vi "TranslatorBooster.vi"() -> ()   [LabVIEW 2014, in "Complex Numbers.lvlib"]
uses:
  <vilib>/Aledyne-TSXperts/Arduino Compatible Compiler for LabVIEW/addons/Complex Numbers/Complex Numbers.lvlib
  <vilib>/regexp/Match Regular Expression.xnode
panel:
  in  "Output dir":path=path "C:/Program Files/National Instruments/LabVIEW 2014/vi.lib/Aledyne-TSXperts/Arduino Compatible Compiler for LabVIEW/addons/Complex Numbers/generated VIs"
  out "Func. output type":string[](array[string])
  out "Params":string[][](array[string])
  out "Func. params":string[](array[string])
  out "Function actual token":string
  out "Readed functions":string[](array[string])
  out "Function Name":string
  out "Function name reading":bool
  out "Class name found.":bool
  out "Functions beginning found.":bool
  out "Input header file.":string[](array[string])
  out "Class name":string
  out "Error Out":errorcluster
  in  "Error In":errorcluster
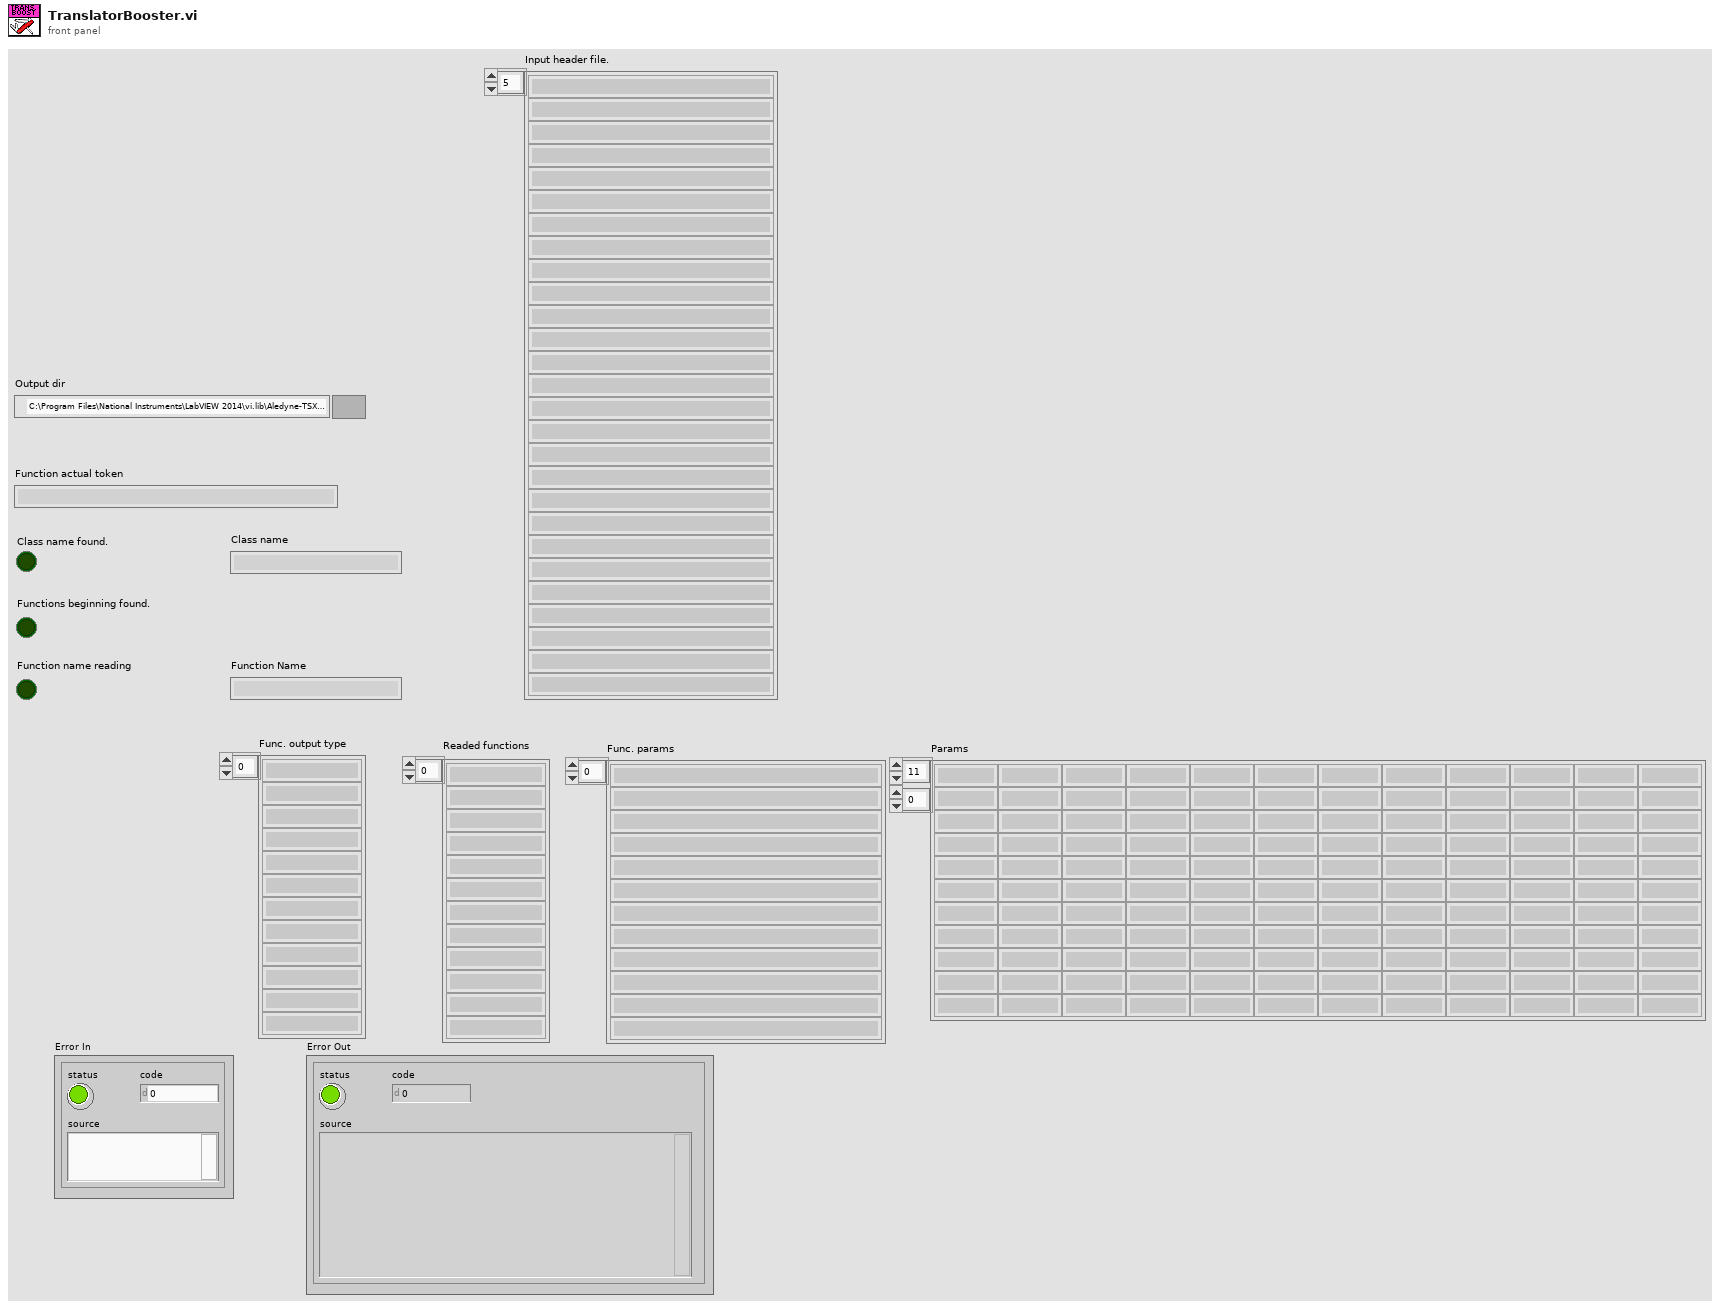
[diagram p1: front panel]
types:
  T1 = enum16{"open", "replace", "create", "open or create", "replace or create", "replace or create with confirmation"}
  T2 = cluster{"Function names":string[], "Function parameters":string[][], "Output types":string[]}
  T3 = enum32{"invalid lock state", "Not Locked", "Locked (No Password)", "Password-protected"}
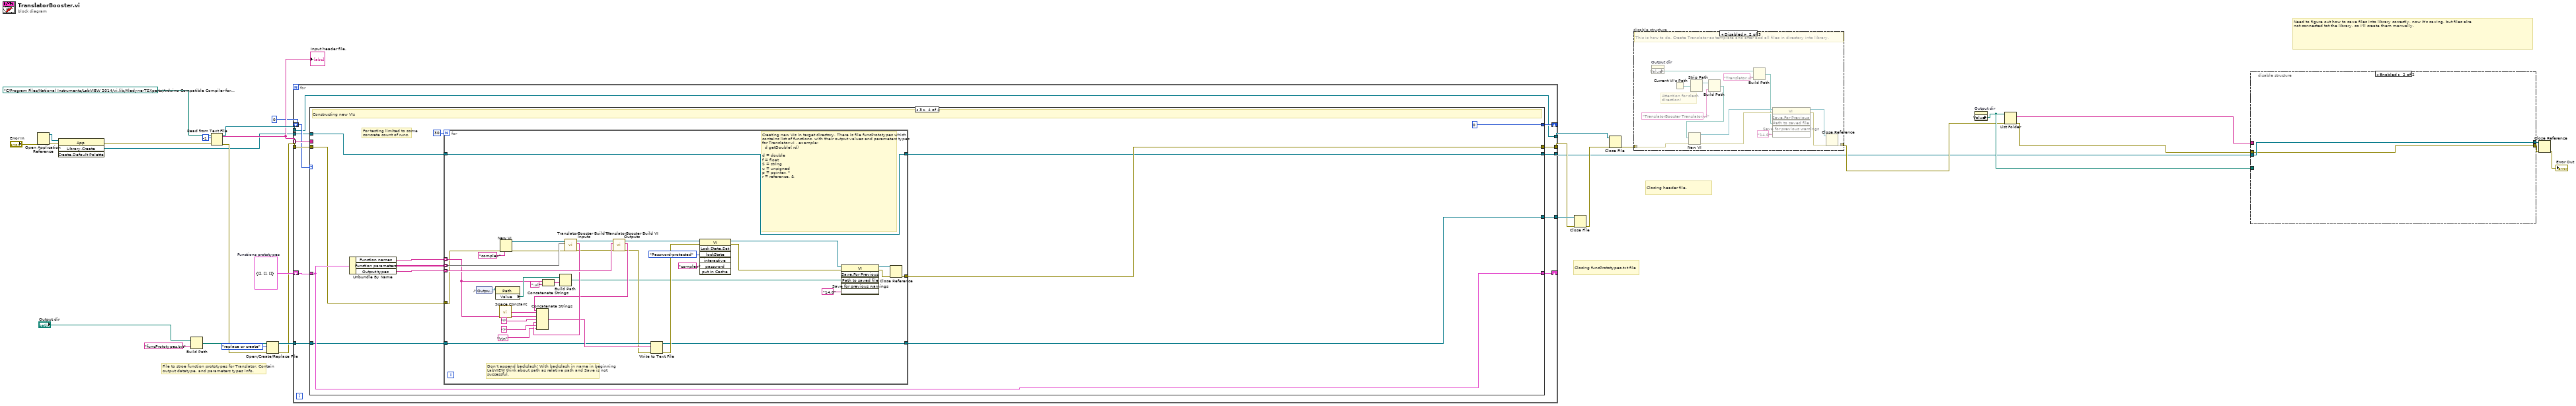
[diagram p0: block diagram]
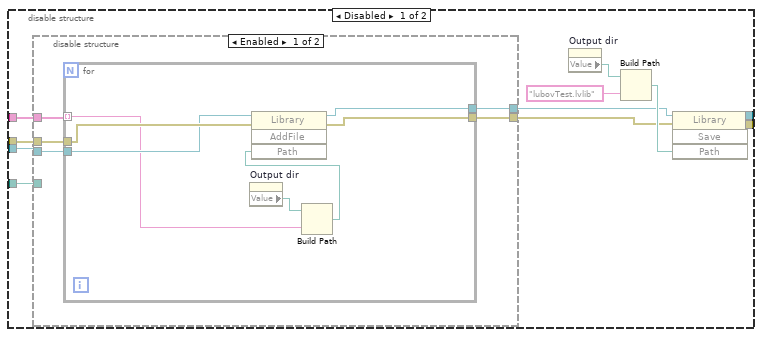
[diagram p2: hidden frame]
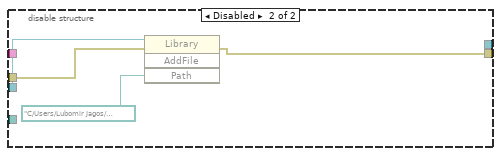
[diagram p3: hidden frame]
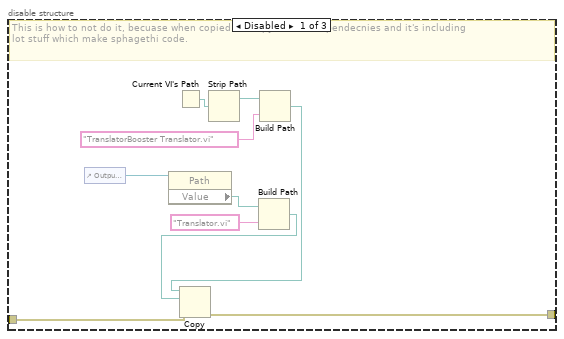
[diagram p4: hidden frame]
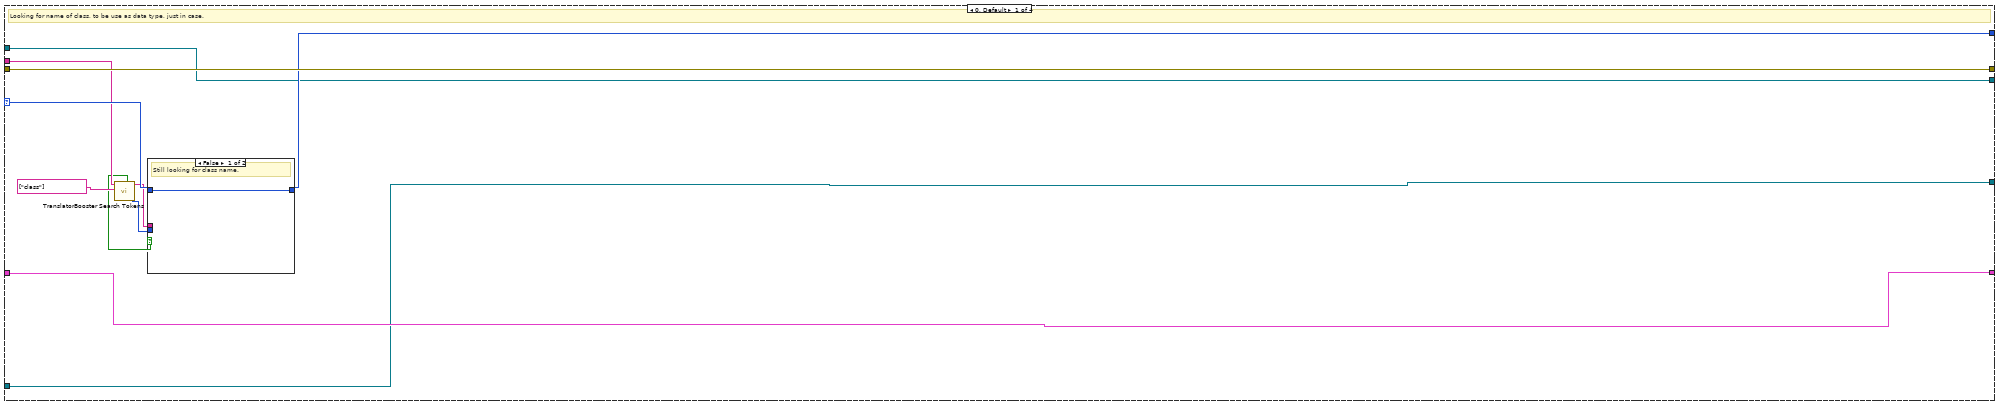
[diagram p6: hidden frame]
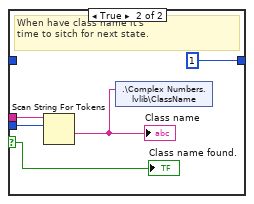
[diagram p7: hidden frame]
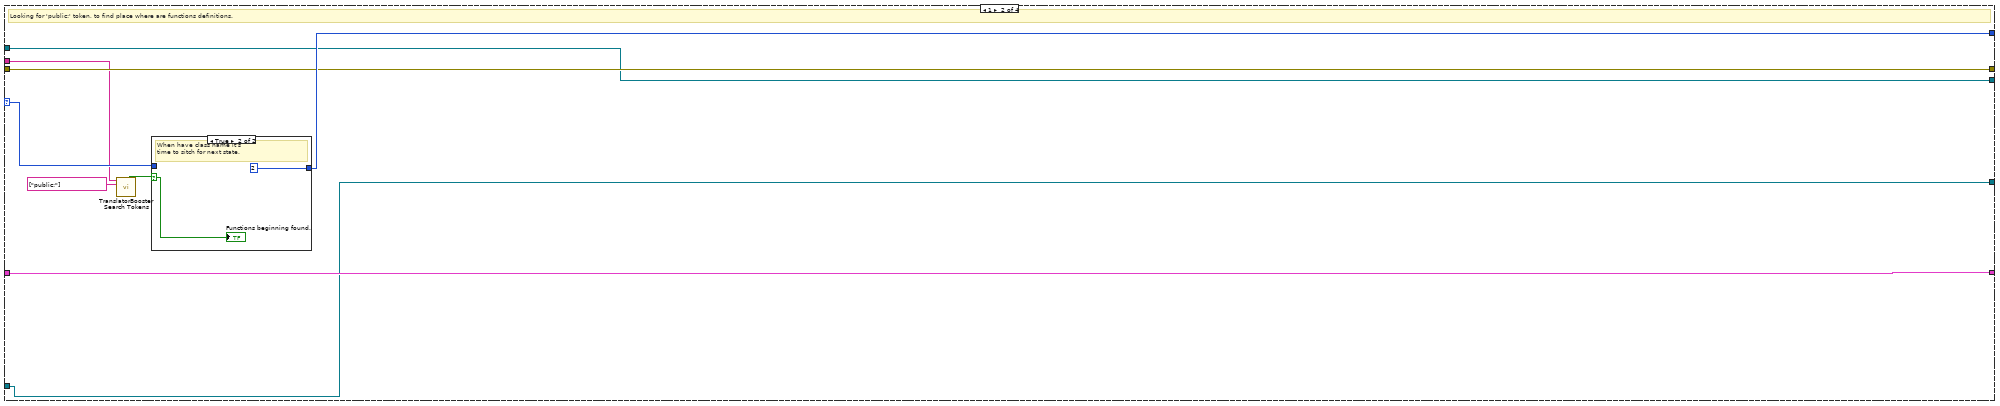
[diagram p8: hidden frame]
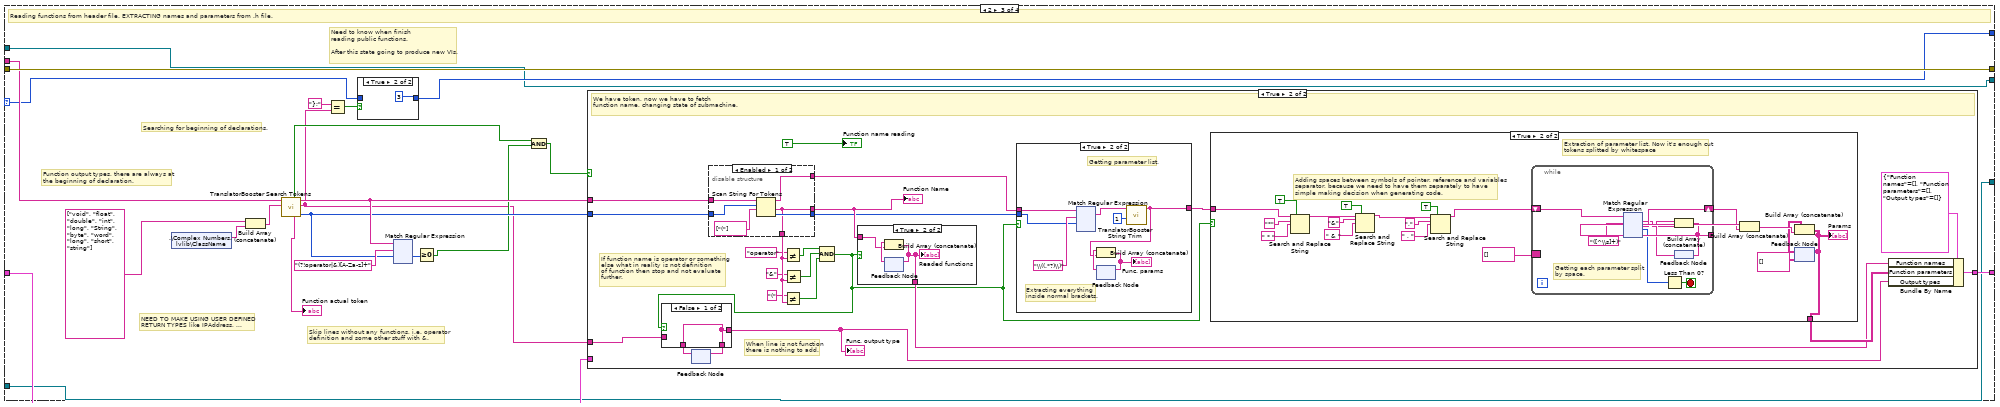
[diagram p10: hidden frame]
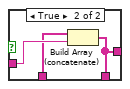
[diagram p13: hidden frame]
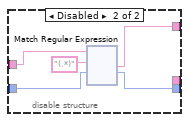
[diagram p16: hidden frame]
diagram:
  w25 = T2 {"Function names"=[], "Function parameters"=[], "Output types"=[]}  # Functions prototypes
  # "Need to figure out how to save files into library correctly, now it's saving, but files alre\nnot connected tot the library, so I'll create them manually."
  # "File to stroe function prototypes for Translator. Contain\noutput datatype, and parameters types info."
  # "Closing header file."
  # "Closing funcPrototypes.txt file"
  n1 = Open Application Reference(8:"Error In") -> (0:w12:errorcluster, 3:w11:refnum<vi>)  [unwired: 3 in]
  n2 = invoke class="App" method="Library.Create"(reference=w11, error in=w12) -> (error out=w9:errorcluster, "Create Library"=w10:refnum<vi>)  [unwired: 2 in, 2 out]
  n3 = Build Path(base path="Output dir", name or relative path="funcPrototypes.txt") -> (appended path=w18:path)
  n4 = Read from Text File(file (use dialog)=path "C:/Program Files/National Instruments/LabVIEW 2014/vi.lib/Aledyne-TSXperts/Arduino Compatible Compiler for LabVIEW/addons/Complex Numbers/libraries/____aux_complex.h", count=-1, error in=w9) -> (refnum out=w28:refnum<file>, text=w27:string[], error out=w17:errorcluster)  [unwired: 1 in, 1 out]
  "Input header file." <- w27
  n5 = Open/Create/Replace File(file path (use dialog)=w18, error in=w17, operation (0:open)=T1."replace or create") -> (refnum out=w23:refnum<file>, error out=w16:errorcluster)  [unwired: 3 in, 1 out]
  n6 = for {
    tunnel: [w38] -> w31
    tunnel: w16 -> [w42]
    tunnel: w28 -> [w38]
    tunnel: w27 -> [w43] mode=indexing
    tunnel: [w41] -> w21
    shift-right: [w40] -> _
    shift-left: 0 ("offset past token") -> [w39]
    shift-right: [w37] -> _
    shift-left: w25 -> [w36]
    tunnel: w23 -> [w35]
    tunnel: [w34] -> w22
    tunnel: w10 -> [w33]
    tunnel: [w32] -> w1
    n7 = case shown="3" w39 {
      selector: w39 -> [w53 w69 w79 _]
      tunnel: w43 -> [w50 w65 w93 _]
      tunnel: w42 -> [w54 w67 w94 w638]
      tunnel: [w54 w67 w94 w636] -> w41
      tunnel: [w52 w68 w78 0 ("offset past token")] -> w40
      tunnel: [w46 w63 w76 w641] -> w37
      tunnel: w36 -> [w46 w63 w75 w641]
      tunnel: w35 -> [w45 w62 w74 w635]
      tunnel: [w45 w62 w74 w634] -> w34
      tunnel: w33 -> [w44 w61 w73 w633]
      tunnel: [w44 w61 w73 w632] -> w32
      frame 0, Default {
        # "Looking for name of class, to be use as data type, just in case."
        n8 = call <vilib>:"TranslatorBooster Search Tokens.vi"("search tokens"=string[] ["class"] ("operators (none)"), "input string"=w50) -> ("offset past token"=w49:i32, "input string"=w47:string, "token found?"=w48:bool)  [unwired: 4 in, 3 out]
        n9 = case shown="False" w48 {
          selector: w48 -> [_ w57]
          tunnel: w49 -> [_ w60]
          tunnel: w47 -> [_ w59]
          tunnel: w53 -> [w55 _]
          tunnel: [w55 1 ("offset past token")] -> w52
          frame False {
            # "Still looking for class name."
          }
          frame True {
            # "When have class name it's\ntime to sitch for next state."
            n10 = Scan String For Tokens(8:w60, 9:w59) -> (1:w56:string)  [unwired: 4 in, 3 out]
            "Class name" <- w56
            n11 = shared-variable ".\\Complex Numbers.lvlib\\ClassName"(w56) -> ()  [unwired: 1 in, 1 out]
            "Class name found." <- w57
          }
        }
      }
      frame 1 {
        # "Looking for 'public:' token, to find place where are functions definitions."
        n12 = call <vilib>:"TranslatorBooster Search Tokens.vi"("search tokens"=string[] ["public:"] ("operators (none)"), "input string"=w65) -> ("token found?"=w64:bool)  [unwired: 4 in, 5 out]
        n13 = case shown="True" w64 {
          selector: w64 -> [_ w71]
          tunnel: [w70 2 ("offset past token")] -> w68
          tunnel: w69 -> [w70 _]
          frame False {
            # "Still looking for functions\nbeginning."
          }
          frame True {
            # "When have class name it's\ntime to sitch for next state."
            "Functions beginning found." <- w71
          }
        }
      }
      frame 2 {
        # "NEED TO MAKE USING USER DEFINED\nRETURN TYPES like IPAddress, ..."
        # "Function output types, there are always at\nthe beginning of declaration."
        # "Need to know when finish\nreading public functions.\n\nAfter this state going to produce new VIs."
        # "Searching for beginning of declarations."
        # "Skip lines without any functions, i.e. operator\ndefinition and some other stuff with &."
        # "Reading functions from header file. EXTRACTING names and parameters from .h file."
        n14 = shared-variable ".\\Complex Numbers.lvlib\\ClassName"() -> (w91:string)  [unwired: 1 in, 1 out]
        n15 = Build Array (concatenate)(string[] ["void", "float", "double", "int", "long", "String", "byte", "word", "long", "short", "string"] ("operators (none)"), w91) -> (w90:string[])
        n16 = call <vilib>:"TranslatorBooster Search Tokens.vi"("search tokens"=w90, "input string"=w93) -> ("offset past token"=w83:i32, "output token"=w77:string, "input string"=w86:string, "actual token"=→"Function actual token":string, "token found?"=w85:bool)  [unwired: 4 in, 1 out]
        n17 = Equal?(x="};", y=w77) -> (x = y?=w80:bool)
        n18 = case shown="True" w80 {
          tunnel: w79 -> [w95 _]
          tunnel: [w95 3 ("offset past token")] -> w78
          frame False {
          }
          frame True {
          }
        }
        n19 = xnode "Match Regular Expression"("input string"=w86, "regular expression"="(?!operator|&)[A-Za-z]+", "offset (0)"=w83) -> ("offset past match"=w88:i32)  [unwired: 3 in, 4 out]
        n20 = Greater Or Equal To 0?(x=w88) -> (x >= 0?=w82:bool)
        n21 = Compound Arithmetic op=AND(w85, w82) -> (w84:bool)
        n22 = case shown="True" w84 {
          tunnel: w86 -> [_ w233]
          tunnel: w83 -> [_ w232]
          tunnel: w77 -> [_ w215]
          tunnel: [w211 w216] -> w76
          tunnel: w75 -> [w211 _]
          frame False {
            # "Still looking for functions\nbeginning."
          }
          frame True {
            # "When line is not function\nthere is nothing to add."
            # "If function name is operator or something\nelse what in reality is not definition\nof function then stop and not evaluate\nfurther."
            # "We have token, now we have to fetch\nfunction name, changing state of submachine."
            n23 = feedback #1() -> (w213:string[])  [unwired: 1 in]
            n24 = disable-structure shown="Enabled" {
              disable-tunnel: w233 -> [w509 w514]
              disable-tunnel: w232 -> [w508 w510]
              disable-tunnel: [w506 w512] -> w231
              disable-tunnel: [w505 w511] -> w228
              disable-tunnel: [w504 _] -> w229
              disable-tunnel: [w504 _] -> w227
              frame Enabled {
                n25 = Scan String For Tokens(7:string[] ["("] ("operators (none)"), 8:w508, 9:w509) -> (0:w505:i32, 1:w504:string, 3:w506:string)  [unwired: 3 in, 1 out]
              }
              frame Disabled {
                n26 = xnode "Match Regular Expression"("input string"=w514, "regular expression"="(.*)", "offset (0)"=w510) -> ("after match"=w512:string, "offset past match"=w511:i32)  [unwired: 3 in, 3 out]
              }
            }
            "Function Name" <- w229
            n27 = Not Equal?(x="operator", y=w227) -> (x != y?=w223:bool)
            n28 = Not Equal?(x="(", y=w227) -> (x != y?=w221:bool)
            n29 = Not Equal?(x="&", y=w227) -> (x != y?=w222:bool)
            n30 = Compound Arithmetic op=AND(w223, w222, w221) -> (w212:bool)
            n31 = case shown="False" w212 {
              tunnel: w215 -> [_ w237]
              tunnel: [w235 w238] -> w219
              tunnel: [w235 w238] -> w214
              tunnel: w213 -> [w235 w236]
              frame False {
              }
              frame True {
                n32 = Build Array (concatenate)(w236, w237) -> (w238:string[])
              }
            }
            "Func. output type" <- w219
            n33 = feedback-in #1(w214) -> ()
            n34 = case shown="True" w212 {
              tunnel: w229 -> [_ w630]
              tunnel: [_ w629] -> w217
              frame False {
              }
              frame True {
                n35 = feedback #2() -> (w631:string[])  [unwired: 1 in]
                n36 = Build Array (concatenate)(w631, w630) -> (w629:string[])
                "Readed functions" <- w629
                n37 = feedback-in #2(w629) -> ()
              }
            }
            n38 = case shown="True" w212 {
              tunnel: w231 -> [w381 w389]
              tunnel: [w381 w386] -> w230
              tunnel: w228 -> [_ w383]
              frame False {
              }
              frame True {
                # "Extracting everything\ninside normal brackets."
                # "Getting parameter list."
                n39 = xnode "Match Regular Expression"("input string"=w389, "regular expression"="\\((.*?)\\)", "offset (0)"=w383) -> ("whole match"=w385:string)  [unwired: 3 in, 4 out]
                n40 = feedback #3() -> (w387:string[])  [unwired: 1 in]
                n41 = call <vilib>:"TranslatorBooster String Trim.vi"("Count"=u8 1, "String In"=w385) -> ("Trimmed String"=w386:string)  [unwired: 9 in]
                n42 = Build Array (concatenate)(w387, w386) -> (w382:string[])
                "Func. params" <- w382
                n43 = feedback-in #3(w382) -> ()
              }
            }
            n44 = case shown="True" w212 {
              tunnel: w230 -> [_ w246]
              tunnel: [_ w252] -> w220
              frame False {
              }
              frame True {
                # "Adding spaces between symbols of pointer, reference and variables\nseparator, because we need to have them separately to have\nsimple making decision when generating code."
                # "Extraction of parameter list. Now it's enough cut\ntokens splitted by whitespace"
                n45 = Search and Replace String(replace all?=TRUE ("replace all? (F)"), input string=w246, search string="*", replace string=" * " ("search string")) -> (result string=w251:string)  [unwired: 4 in, 3 out]
                n46 = Search and Replace String(replace all?=TRUE ("replace all? (F)"), input string=w251, search string="&", replace string=" & " ("search string")) -> (result string=w243:string)  [unwired: 4 in, 3 out]
                n47 = Search and Replace String(replace all?=TRUE ("replace all? (F)"), input string=w243, search string=",", replace string=" , " ("search string")) -> (result string=w242:string)  [unwired: 4 in, 3 out]
                n48 = while {
                  tunnel: [w265] -> w257
                  border: string[] [] -> [_]
                  shift-right: [w263] -> w254
                  shift-left: w242 -> [w259]
                  stop <- w266 stop-if-true
                  # "Getting each parameter split\nby space."
                  n49 = xnode "Match Regular Expression"("input string"=w259, "regular expression"="([^\\s]+)") -> ("whole match"=w260:string, "after match"=w263:string, "offset past match"=w262:i32)  [unwired: 4 in, 2 out]
                  n50 = Less Than 0?(x=w262) -> (x < 0?=w266:bool)
                  n51 = feedback #4() -> (w261:string[])
                  n52 = Build Array (concatenate)(w261, w260) -> (w265:string[])
                  n53 = feedback-in #4(w265) -> ()
                }
                n54 = Build Array (concatenate)(w257, w254) -> (w256:string[])
                n55 = feedback #5(string[][] []) -> (w255:string[][])
                n56 = Build Array (concatenate)(w255, w256) -> (w252:string[][])
                "Params" <- w252
                n57 = feedback-in #5(w252) -> ()
              }
            }
            n58 = Bundle By Name(cluster=T2 {"Function names"=[], "Function parameters"=[], "Output types"=[]} ("input cluster"), "Function names"=w217, "Function parameters"=w220, "Output types"=w219) -> (w216:T2)
            "Function name reading" <- TRUE ("Function return type reading")
          }
        }
      }
      frame 3 {
        # "For testing limited to some\nconcrete count of runs."
        # "Constructing new VIs"
        n59 = Unbundle By Name(w641) -> ("Function names"=w643:string[], "Function parameters"=w640:string[][], "Output types"=w639:string[])
        n60 = for {
          N: 30 -> [_]
          tunnel: w643 -> [w658] mode=indexing
          tunnel: w640 -> [w677] mode=indexing
          tunnel: w639 -> [w676] mode=indexing
          tunnel: w638 -> [w653]
          tunnel: [w652] -> w636
          tunnel: w635 -> [w666]
          tunnel: [w662] -> w634
          tunnel: w633 -> [w644]
          tunnel: [w644] -> w632
          # "Don't append backslash! With backslash in name in beginning\nLabVIEW think about path as relative path and Save is not\nsuccessful."
          # "Creating new VIs in target directory. There is file funcPrototypes which contains list of functions, with their output values and parameters types for Translator.vi , example:\n  d getDouble( rd)\n\nd = double\nf = float\nS = string\nu = unsigned\np = pointer, *\nr = reference, &"
          n61 = control-ref of="Output dir"() -> (w661:refnum<vi>)
          n62 = property class="Path"(reference=w661) -> ("Value"=w660:path)  [unwired: 1 in, 2 out]
          n63 = call <vilib>:"Space Constant.vi"() -> ("String"=w669:string)
          n64 = New VI(6:"complex" ("password"), 8:w653) -> (0:w656:errorcluster, 3:w648:refnum<vi>)  [unwired: 5 in]
          n65 = Concatenate Strings(w658, ".vi" ("string")) -> (w659:string)
          n66 = Build Path(base path=w660, name or relative path=w659) -> (appended path=w651:path)
          n67 = call <vilib>:"TranslatorBooster Build VI Inputs.vi"("error in (no error)"=w656, "Function parameters"=w677, "VI in"=w648) -> ("error out"=w655:errorcluster, "ParamsType abbr."=w670:string, "VI out"=w654:refnum<vi>)  [unwired: 6 in]
          n68 = call <vilib>:"TranslatorBooster Build VI Outputs.vi"("error in (no error)"=w655, "Output type"=w676, "VI in"=w654) -> ("error out"=w665:errorcluster, "OutputType abbr."=w668:string, "VI out"=w675:refnum<vi>)  [unwired: 6 in]
          n69 = Concatenate Strings(w668, w669, w658, "(" ("string"), w670, ")" ("string"), "\r\n") -> (w667:string)
          n70 = Write to Text File(file (use dialog)=w666, text=w667, error in=w665) -> (refnum out=w662:refnum<file>, error out=w664:errorcluster)  [unwired: 1 in, 1 out]
          n71 = invoke class="VI" method="Lock State.Set"(reference=w675, error in=w664, "lockState"=T3."Password-protected" ("Lock State"), "password"="complex" ("Password")) -> (reference out=w645:refnum<vi>, error out=w646:errorcluster)  [unwired: 3 in, 5 out]
          n72 = invoke class="VI" method="Save.For Previous"(reference=w645, error in=w646, "Path to saved file"=w651, "Oldest compatible target version"="14.0" ("Target Version")) -> (reference out=w650:refnum<vi>, error out=w649:errorcluster)  [unwired: 2 in, 4 out]
          n73 = Close Reference(reference=w650, error in (no error)=w649) -> (error out=w652:errorcluster)
        }
      }
    }
  }
  n74 = Close File(refnum=w22, error in=w21) -> (error out=w20:errorcluster)  [unwired: 1 out]
  n75 = Close File(refnum=w31, error in=w20) -> (error out=w14:errorcluster)  [unwired: 1 out]
  n76 = disable-structure shown="Disabled" {
    disable-tunnel: w14 -> [w688 w702 w703]
    disable-tunnel: [w679 w695 w703] -> w6
    frame Disabled {
      # "This is how to not do it, becuase when copied it's copy with all dependecnies and it's including\nlot stuff which make sphagethi code."
      n77 = control-ref of="Output dir"() -> (w682:refnum<vi>)
      n78 = property class="Path"(reference=w682) -> ("Value"=w681:path)  [unwired: 1 in, 2 out]
      n79 = Current VI's Path() -> (path=w687:path)
      n80 = Strip Path(path=w687) -> (stripped path=w686:path)  [unwired: 1 out]
      n81 = Build Path(base path=w681, name or relative path="Translator.vi") -> (appended path=w680:path)
      n82 = Build Path(base path=w686, name or relative path="TranslatorBooster Translator.vi") -> (appended path=w684:path)
      n83 = Copy(8:w688, 10:w680, 11:w684) -> (0:w679:errorcluster)  [unwired: 2 in, 2 out]
    }
    frame Disabled {
      # "Attention for slash\ndirection!"
      # "This is how to do. Create Translator as template and after add all files in directory into library."
      n84 = property on="Output dir" class="Path"() -> ("Value"=w691:path)  [unwired: 2 in, 2 out]
      n85 = Current VI's Path() -> (path=w689:path)
      n86 = Strip Path(path=w689) -> (stripped path=w690:path)  [unwired: 1 out]
      n87 = Build Path(base path=w690, name or relative path="TranslatorBooster Translator.vi") -> (appended path=w698:path)
      n88 = New VI(8:w702, 10:w698) -> (0:w700:errorcluster, 3:w701:refnum<vi>)  [unwired: 5 in]
      n89 = Build Path(base path=w691, name or relative path="Translator.vi") -> (appended path=w696:path)
      n90 = invoke class="VI" method="Save.For Previous"(reference=w701, error in=w700, "Path to saved file"=w696, "Oldest compatible target version"="14.0" ("Target Version")) -> (reference out=w693:refnum<vi>, error out=w694:errorcluster)  [unwired: 2 in, 4 out]
      n91 = Close Reference(reference=w693, error in (no error)=w694) -> (error out=w695:errorcluster)
    }
    frame Enabled {
    }
  }
  n92 = property on="Output dir" class="Path"() -> ("Value"=w7:path)  [unwired: 2 in, 2 out]
  n93 = List Folder(path=w7, error in=w6) -> (filenames=w8:string[], error out=w2:errorcluster)  [unwired: 2 in, 2 out]
  n94 = disable-structure shown="Enabled" {
    disable-tunnel: w8 -> [w714 _]
    disable-tunnel: w7 -> [w713 _]
    disable-tunnel: [w712 w733] -> w4
    disable-tunnel: [w711 w732] -> w3
    disable-tunnel: w2 -> [w710 w732]
    disable-tunnel: w1 -> [w709 w733]
    frame Disabled {
      n95 = disable-structure shown="Enabled" {
        disable-tunnel: w714 -> [w719 _]
        disable-tunnel: w710 -> [w717 w728]
        disable-tunnel: w709 -> [w718 w730]
        disable-tunnel: w713 -> [_ _]
        disable-tunnel: [w716 w731] -> w705
        disable-tunnel: [w715 _] -> w704
        frame Enabled {
          n96 = for {
            tunnel: w719 -> [w721] mode=indexing
            tunnel: w718 -> [w724]
            tunnel: w717 -> [w725]
            tunnel: [w723] -> w716
            tunnel: [w722] -> w715
            n97 = property on="Output dir" class="Path"() -> ("Value"=w726:path)  [unwired: 2 in, 2 out]
            n98 = Build Path(base path=w726, name or relative path=w721) -> (appended path=w720:path)
            n99 = invoke class="Library" method="AddFile"(reference=w724, error in=w725, "Path"=w720) -> (reference out=w722:refnum<vi>, error out=w723:errorcluster)  [unwired: 1 in, 2 out]
          }
        }
        frame Disabled {
          n100 = invoke class="Library" method="AddFile"(reference=w730, error in=w728, "Path"=path "C:/Users/Lubomir Jagos/Documents/LabView/Arduino_projects/Blink.vi") -> (reference out=w727:refnum<vi>, error out=w731:errorcluster)  [unwired: 1 in, 2 out]
        }
      }
      n101 = property on="Output dir" class="Path"() -> ("Value"=w708:path)  [unwired: 2 in, 2 out]
      n102 = Build Path(base path=w708, name or relative path="lubovTest.lvlib" ("string")) -> (appended path=w706:path)
      n103 = invoke class="Library" method="Save"(reference=w704, error in=w705, "Path"=w706) -> (reference out=w712:refnum<vi>, error out=w711:errorcluster)  [unwired: 1 in, 2 out]
    }
    frame Enabled {
    }
  }
  n104 = Close Reference(reference=w4, error in (no error)=w3) -> (error out=→"Error Out":errorcluster)
